vi "python_test.vi"() -> ()   [LabVIEW 2021]
panel:
  out "Output":string
  in  "Order":i32
  out "Python error":errorcluster={"status"=FALSE, "code"=200012, "source"="DAQmx Control Task.vi:3900001"}
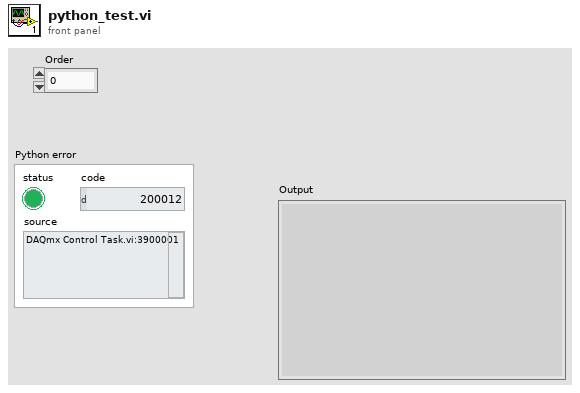
[diagram p1: front panel]
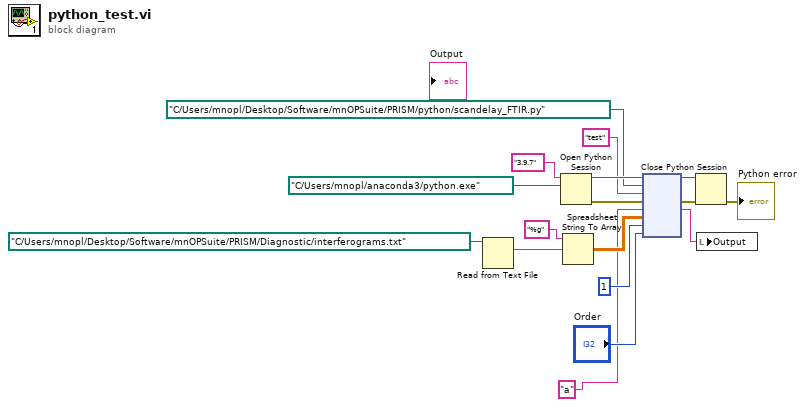
[diagram p0: block diagram]
diagram:
  n1 = Read from Text File(file (use dialog)=path "C:/Users/mnopl/Desktop/Software/mnOPSuite/PRISM/Diagnostic/interferograms.txt") -> (text=w7:string)  [unwired: 3 in, 3 out]
  n2 = Open Python Session(python version="3.9.7", python path=path "C:/Users/mnopl/anaconda3/python.exe") -> (session out=w15:refnum<k35>, error out=w12:errorcluster)  [unwired: 1 in]
  n3 = Spreadsheet String To Array(format string="%g", spreadsheet string=w7) -> (array=w8:dbl[][])  [unwired: 2 in]
  n4 = node(w15, path "C:/Users/mnopl/Desktop/Software/mnOPSuite/PRISM/python/scandelay_FTIR.py", "test", w12, "a", w8, 1, "Order") -> (w9:refnum<k35>, w11:errorcluster, w4:string)  [unwired: 3 in, 2 out]
  n5 = Close Python Session(session in=w9, error in=w11) -> (11:→"Python error":errorcluster)
  n6 = local write "Output"(w4) -> ()
